vi "Img Clear Image.vi"(8 "error in (no error)":errorcluster, 11 "LF2R IDE in":refnum<class "Main Panel.lvclass">) -> (0 "error out":errorcluster, 3 "LF2R IDE out":refnum<class "Main Panel.lvclass">)   [LabVIEW 2018, in "Main Panel.lvlib" / "Main Panel.lvclass"]
uses:
  Main Panel.lvclass
  Main Panel.lvclass/Main Panel.ctl
  Image/Image Process.lvclass
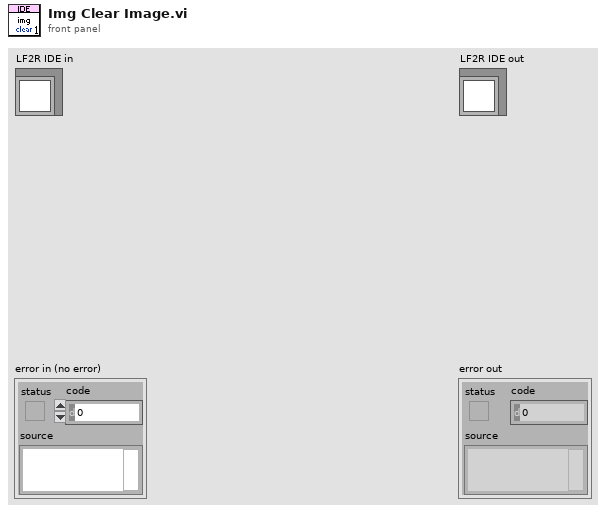
[diagram p1: front panel]
types:
  T1 = typedef "Image Type" = u32
  T2 = typedef "IMAQ Image.ctl" = refnum<image>
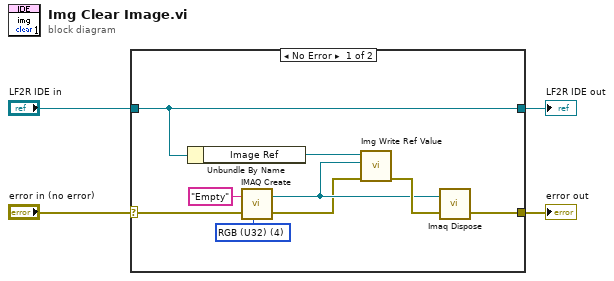
[diagram p0: block diagram]
diagram:
  n1 = case shown="No Error" "error in (no error)" {
    selector: "error in (no error)" -> [w6 w15]
    tunnel: [w5 w15] -> w3
    tunnel: [w7 w14] -> w1
    tunnel: "LF2R IDE in" -> [w7 w14]
    frame No Error {
      w12 = T1 4 items=["Grayscale (U8)", "Grayscale (I16)", "Grayscale (SGL)", "Complex (CSG)", "RGB (U32)", "HSL (U32)", "RGB (U64)", "Grayscale (U16)"] ("Image Type")
      n2 = Unbundle By Name(w7) -> ("Image Ref"=w8:refnum<vi>)
      n3 = call "IMAQ Create"("Image Name"="Empty", "Image Type"=w12, "error in (no error)"=w6) -> ("New Image"=w10:T2, "error out"=w9:errorcluster)  [unwired: 2 in]
      n4 = call "Img Write Ref Value.vi"("error in (no error)"=w9, "Image"=w10, "Image Ref"=w8) -> ("error out"=w11:errorcluster)  [unwired: 8 in]
      n5 = call "Imaq Dispose"("Image"=w10, "error in (no error)"=w11) -> ("error out"=w5:errorcluster)  [unwired: 4 in]
    }
    frame Error {
    }
  }
  "error out" <- w3
  "LF2R IDE out" <- w1
